vi "sub_pf_localization.vi"(11 "p-val out":T2) -> ()   [LabVIEW 2019]
uses:
  <vilib>/Analysis/Matrix/Datatypes/RealMatrix.ctl
  Ctrl/cmd_common.ctl
  <vilib>/Analysis/baseanly.llb/Real A x B.vi
  <vilib>/ptbypt/NI_PtbyPt.lvlib
  <vilib>/Analysis/NI_AALBase.lvlib
  <vilib>/Analysis/Matrix/NI_Matrix.lvlib
panel:
  out "x":T1 caption="전치 행렬"
  out "px":T1
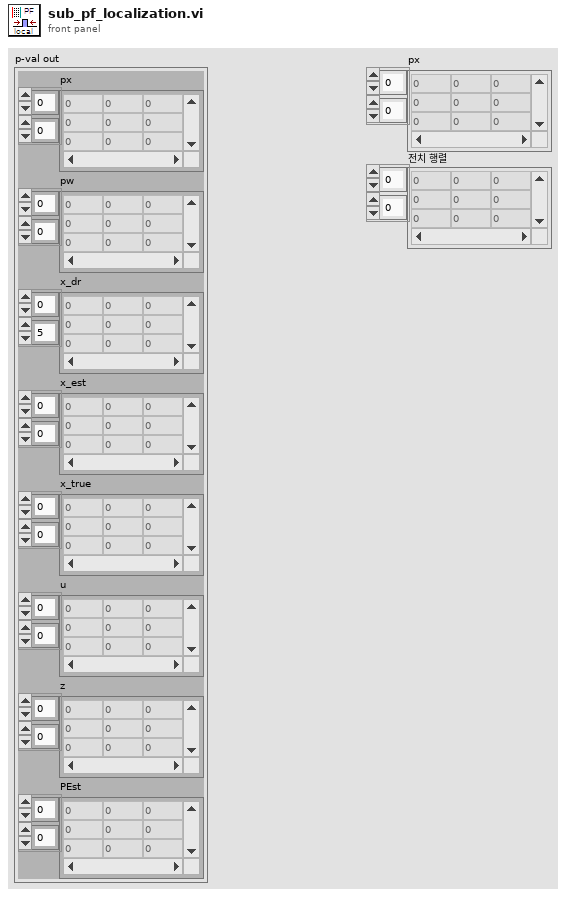
[diagram p1: front panel]
types:
  T1 = typedef "NI_Matrix.lvlib/RealMatrix.ctl" = dbl[][]
  T2 = cluster{"px":T1, "pw":T1, "x_dr":T1, "x_est":T1, "x_true":T1, "u":T1, "z":T1, "PEst":T1}
  T3 = typedef "cmd_common.ctl" = enum16{"read", "write"}
  T4 = cluster{"DT":dbl, "SIM_TIME":dbl, "MAX_RANGE":dbl, "NP":u32, "NTh":u32, "Q":T1, "R":T1, "Q_sim":T1, "R_sim":T1, "rf_id":cluster{"x":dbl, "y":dbl}[]}
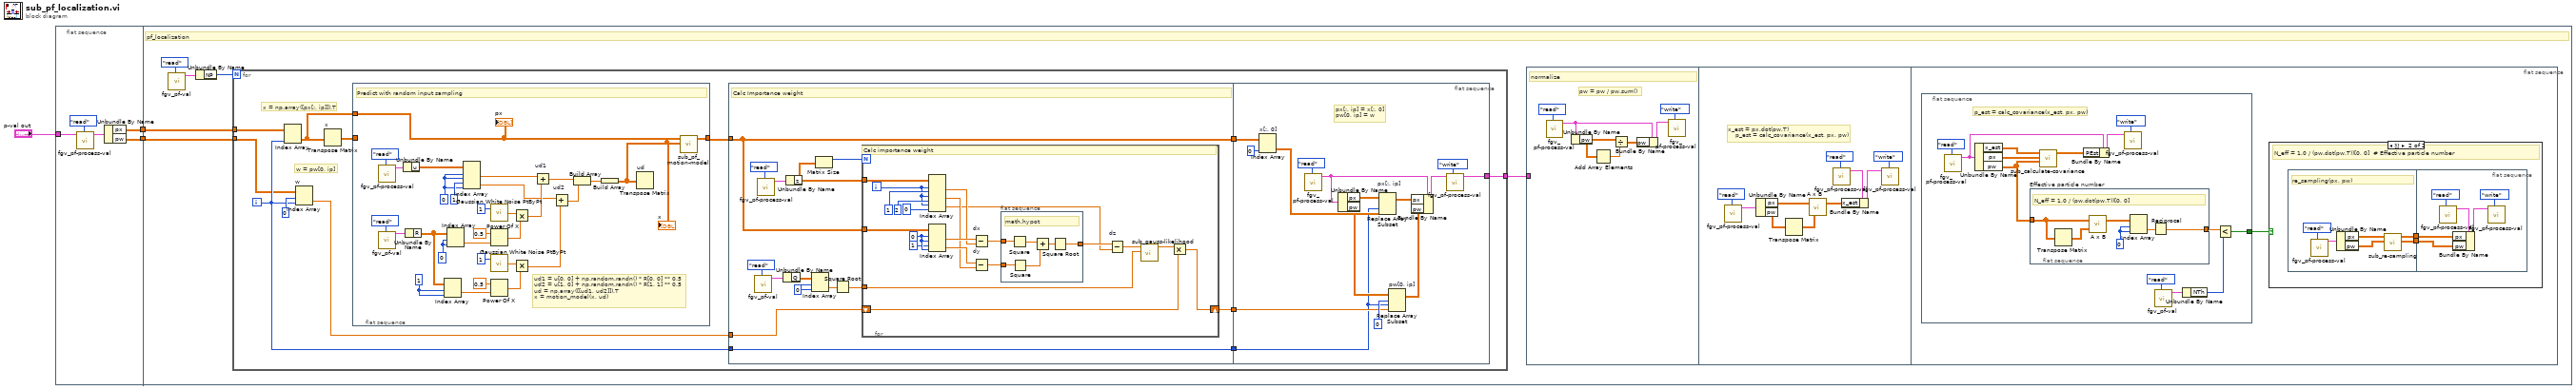
[diagram p0: block diagram]
diagram:
  n1 = flat-sequence {
    tunnel: [w6] -> w3
    tunnel: [w5] -> w2
    tunnel: "p-val out" -> [w4]
    tunnel: w3 -> [w10]
    tunnel: w2 -> [w9]
    frame #0 {
      n2 = call "fgv_pf-process-val.vi"("cmd"=cmd_common."read", "p-val"=w4) -> ("p-val out"=w8:T2)  [unwired: 9 in]
      n3 = Unbundle By Name(w8) -> ("px"=w6:T1, "pw"=w5:T1)
    }
    frame #1 {
      # "pf_localization"
      n4 = call "fgv_pf-val.vi"("cmd"=cmd_common."read") -> ("pf-val out"=w13:T4)  [unwired: 10 in]
      n5 = Unbundle By Name(w13) -> ("NP"=w11:u32)
      n6 = for {
        N: w11 -> [_]
        tunnel: [w71] -> w14
        tunnel: w10 -> [w68]
        tunnel: w9 -> [w67]
        i -> [w70]
        # "x = np.array([px[:, ip]]).T"
        # "w = pw[0, ip]"
        n7 = Index Array(array=w68, index (col)=w70) -> (element=w66:T1)  [unwired: 1 in]
        n8 = Index Array "w"(array=w67, index (row)=0 ("인덱스 (행)"), index (col)=w70) -> (element=w75:dbl)
        n9 = Transpose Matrix "x"(1:w66) -> (0:w69:T1)
        n10 = flat-sequence {
          tunnel: w69 -> [_]
          tunnel: [w80] -> w76
          tunnel: w66 -> [w79]
          frame #0 {
            w88 = 1 ("인덱스 (행)")
            w99 = 0 ("인덱스 (행)")
            w103 = 0 ("인덱스 (행)")
            # "ud1 = u[0, 0] + np.random.randn() * R[0, 0] ** 0.5\nud2 = u[1, 0] + np.random.randn() * R[1, 1] ** 0.5\nud = np.array([[ud1, ud2]]).T\nx = motion_model(x, ud)"
            # "Predict with random input sampling"
            n11 = call "fgv_pf-process-val.vi"("cmd"=cmd_common."read") -> ("p-val out"=w106:T2)  [unwired: 10 in]
            n12 = call "fgv_pf-val.vi"("cmd"=cmd_common."read") -> ("pf-val out"=w100:T4)  [unwired: 10 in]
            n13 = Unbundle By Name(w106) -> ("u"=w105:T1)
            n14 = Unbundle By Name(w100) -> ("R"=w81:T1)
            n15 = Index Array(array=w81, index (row)=w88, index (col)=w88) -> (element=w89:dbl)
            n16 = Index Array(array=w81, index (row)=w99, index (col)=w99) -> (element=w98:dbl)
            n17 = Index Array(array=w105, index (row) #1=w103, index (col) #1=w103, index (row) #2=1 ("인덱스 (행)"), index (col) #2=w103) -> (element #1=w93:dbl, element #2=w86:dbl)
            n18 = call <vilib>:"Gaussian White Noise PtByPt.vi"("standard deviation"=1 ("samples")) -> ("Gaussian white noise"=w95:dbl)  [unwired: 2 in]
            n19 = Power Of X(1:w98, 2:0.5 ("y")) -> (0:w96:dbl)
            n20 = call <vilib>:"Gaussian White Noise PtByPt.vi"("standard deviation"=1 ("samples")) -> ("Gaussian white noise"=w92:dbl)  [unwired: 2 in]
            n21 = Power Of X(1:w89, 2:0.5 ("y")) -> (0:w91:dbl)
            n22 = Multiply(x=w95, y=w96) -> (x*y=w94:dbl)
            n23 = Multiply(x=w92, y=w91) -> (x*y=w85:dbl)
            n24 = Add "ud1"(x=w93, y=w94) -> (x+y=w82:dbl)
            n25 = Add "ud2"(x=w86, y=w85) -> (x+y=w83:dbl)
            n26 = Build Array(w82, w83) -> (w84:dbl[])
            n27 = Build Array(w84) -> (w78:T1)
            "x" <- w78
            n28 = Transpose Matrix "ud"(1:w78) -> ()  [unwired: 1 out]
            n29 = call "sub_pf_motion-model.vi"("u"=w78, "x_true"=w79) -> ("x_true out"=w80:T1)  [unwired: 9 in]
            "px" <- w79
          }
        }
        n30 = flat-sequence {
          tunnel: w76 -> [w109]
          tunnel: w75 -> [w111]
          tunnel: w70 -> [w110]
          tunnel: [w110] -> w74
          tunnel: [w109] -> w73
          tunnel: [w108] -> w72
          tunnel: w72 -> [w153]
          tunnel: w73 -> [w159]
          tunnel: w74 -> [w152]
          tunnel: [w151] -> w71
          frame #0 {
            w114 = 0 ("인덱스 (행)")
            # "Calc Importance weight"
            n31 = call "fgv_pf-val.vi"("cmd"=cmd_common."read") -> ("pf-val out"=w116:T4)  [unwired: 10 in]
            n32 = call "fgv_pf-process-val.vi"("cmd"=cmd_common."read") -> ("p-val out"=w120:T2)  [unwired: 10 in]
            n33 = Unbundle By Name(w116) -> ("Q"=w115:T1)
            n34 = Unbundle By Name(w120) -> ("z"=w118:T1)
            n35 = Index Array(array=w115, index (row)=w114, index (col)=w114) -> (element=w113:dbl)
            n36 = Matrix Size(0:w118) -> (1:w119:i32)  [unwired: 1 out]
            n37 = Square Root(x=w113) -> (sqrt(x)=w112:dbl)
            n38 = for {
              N: w119 -> [_]
              tunnel: w109 -> [w142]
              tunnel: w118 -> [w139]
              tunnel: w112 -> [w126]
              shift-right: [w122] -> w108
              shift-left: w111 -> [w123]
              i -> [w125]
              w141 = 0 ("인덱스 (행)")
              # "Calc importance weight"
              n39 = Index Array(array=w139, index (row) #1=w125, index (col) #1=1 ("인덱스 (열)"), index (row) #2=w125, index (col) #2=2 ("인덱스 (열)"), index (row) #3=w125, index (col) #3=0 ("인덱스 (열)")) -> (element #1=w135:dbl, element #2=w133:dbl, element #3=w128:dbl)
              n40 = Index Array(array=w142, index (row) #1=w141, index (col) #1=w141, index (row) #2=1 ("인덱스 (행)"), index (col) #2=w141) -> (element #1=w136:dbl, element #2=w134:dbl)
              n41 = Subtract "dx"(x=w136, y=w135) -> (x-y=w131:dbl)
              n42 = Subtract "dy"(x=w134, y=w133) -> (x-y=w132:dbl)
              n43 = flat-sequence {
                tunnel: w132 -> [w148]
                tunnel: w131 -> [w147]
                tunnel: [w143] -> w129
                frame #0 {
                  # "math.hypot"
                  n44 = Square(x=w147) -> (x^2=w145:dbl)
                  n45 = Square(x=w148) -> (x^2=w144:dbl)
                  n46 = Add(x=w145, y=w144) -> (x+y=w146:dbl)
                  n47 = Square Root(x=w146) -> (sqrt(x)=w143:dbl)
                }
              }
              n48 = Subtract "dz"(x=w129, y=w128) -> (x-y=w127:dbl)
              n49 = call "sub_gauss-likelihood.vi"("sigma"=w126, "x"=w127) -> ("p"=w124:dbl)  [unwired: 9 in]
              n50 = Multiply ("Multiply.vi")(x=w124, y=w123) -> (x*y=w122:dbl)
            }
          }
          frame #1 {
            # "px[:, ip] = x[:, 0]\npw[0, ip] = w"
            n51 = Index Array "x[:, 0]"(array=w159, index (col)=0) -> (element=w156:T1)  [unwired: 1 in]
            n52 = call "fgv_pf-process-val.vi"("cmd"=cmd_common."read") -> ("p-val out"=w160:T2)  [unwired: 10 in]
            n53 = Unbundle By Name(w160) -> ("px"=w157:T1, "pw"=w155:T1)
            n54 = Replace Array Subset "px[:, ip]"(array=w157, new element=w156, index (col)=w152) -> (w149:T1)  [unwired: 1 in]
            n55 = Replace Array Subset "pw[0, ip]"(array=w155, new element=w153, index (row)=0 ("index (col)"), index (col)=w152) -> (w150:T1)
            n56 = Bundle By Name(cluster=w160, "px"=w149, "pw"=w150) -> (w163:T2)
            n57 = call "fgv_pf-process-val.vi"("cmd"=cmd_common."write", "p-val"=w163) -> ("p-val out"=w151:T2)  [unwired: 9 in]
          }
        }
      }
      n58 = flat-sequence {
        tunnel: w14 -> [_]
        frame #0 {
          # "pw = pw / pw.sum()"
          # "normalize"
          n59 = call "fgv_pf-process-val.vi"("cmd"=cmd_common."read") -> ("p-val out"=w20:T2)  [unwired: 10 in]
          n60 = Unbundle By Name(w20) -> ("pw"=w18:T1)
          n61 = Add Array Elements(numeric array=w18) -> (sum=w17:dbl)
          n62 = Divide(x=w18, y=w17) -> (x/y=w19:T1)
          n63 = Bundle By Name(cluster=w20, "pw"=w19) -> (w21:T2)
          n64 = call "fgv_pf-process-val.vi"("cmd"=cmd_common."write", "p-val"=w21) -> ()  [unwired: 9 in, 1 out]
        }
        frame #1 {
          # "x_est = px.dot(pw.T)\n    p_est = calc_covariance(x_est, px, pw)"
          n65 = call "fgv_pf-process-val.vi"("cmd"=cmd_common."read") -> ("p-val out"=w31:T2)  [unwired: 10 in]
          n66 = Unbundle By Name(w31) -> ("px"=w30:T1, "pw"=w29:T1)
          n67 = Transpose Matrix(1:w29) -> (0:w28:T1)
          n68 = call-poly <vilib>:"A x B.vi"("B"=w28, "A"=w30) -> ("A x B"=w25:T1)  [unwired: 1 out]
          n69 = call "fgv_pf-process-val.vi"("cmd"=cmd_common."read") -> ("p-val out"=w26:T2)  [unwired: 10 in]
          n70 = Bundle By Name(cluster=w26, "x_est"=w25) -> (w27:T2)
          n71 = call "fgv_pf-process-val.vi"("cmd"=cmd_common."write", "p-val"=w27) -> ()  [unwired: 9 in, 1 out]
        }
        frame #2 {
          n72 = flat-sequence {
            tunnel: [w37] -> w32
            frame #0 {
              # "p_est = calc_covariance(x_est, px, pw)"
              n73 = call "fgv_pf-process-val.vi"("cmd"=cmd_common."read") -> ("p-val out"=w35:T2)  [unwired: 10 in]
              n74 = Unbundle By Name(w35) -> ("x_est"=w43:T1, "px"=w44:T1, "pw"=w42:T1)
              n75 = flat-sequence "Effective particle number" {
                tunnel: w42 -> [w51]
                tunnel: [w46] -> w40
                frame #0 {
                  w48 = 0 ("index (row)")
                  # "N_eff = 1.0 / (pw.dot(pw.T))[0, 0]"
                  n76 = Transpose Matrix(1:w51) -> (0:w50:T1)
                  n77 = call-poly <vilib>:"A x B.vi"("B"=w50, "A"=w51) -> ("A x B"=w49:T1)  [unwired: 1 out]
                  n78 = Index Array(array=w49, index (row)=w48, index (col)=w48) -> (element=w47:dbl)
                  n79 = Reciprocal(x=w47) -> (1/x=w46:dbl)
                }
              }
              n80 = call "sub_calculate-covariance.vi"("pw"=w42, "px"=w44, "x_est"=w43) -> ("cov out"=w34:T1)  [unwired: 8 in]
              n81 = Bundle By Name(cluster=w35, "PEst"=w34) -> (w33:T2)
              n82 = call "fgv_pf-process-val.vi"("cmd"=cmd_common."write", "p-val"=w33) -> ()  [unwired: 9 in, 1 out]
              n83 = call "fgv_pf-val.vi"("cmd"=cmd_common."read") -> ("pf-val out"=w39:T4)  [unwired: 10 in]
              n84 = Unbundle By Name(w39) -> ("NTh"=w38:u32)
              n85 = Less?(x=w40, y=w38) -> (x < y?=w37:bool)
            }
          }
          n86 = case shown="참" w32 {
            frame False {
            }
            frame True {
              # "N_eff = 1.0 / (pw.dot(pw.T))[0, 0]  # Effective particle number"
              n87 = flat-sequence {
                tunnel: [w55] -> w53
                tunnel: [w54] -> w52
                tunnel: w53 -> [w63]
                tunnel: w52 -> [w62]
                frame #0 {
                  # "re_sampling(px, pw)"
                  n88 = call "fgv_pf-process-val.vi"("cmd"=cmd_common."read") -> ("p-val out"=w59:T2)  [unwired: 10 in]
                  n89 = Unbundle By Name(w59) -> ("px"=w56:T1, "pw"=w57:T1)
                  n90 = call "sub_re-sampling.vi"("pw"=w57, "px"=w56) -> ("A + c"=w54:T1, "Real Matrix"=w55:T1)  [unwired: 8 in]
                }
                frame #1 {
                  n91 = call "fgv_pf-process-val.vi"("cmd"=cmd_common."read") -> ("p-val out"=w65:T2)  [unwired: 10 in]
                  n92 = Bundle By Name(cluster=w65, "px"=w63, "pw"=w62) -> (w64:T2)
                  n93 = call "fgv_pf-process-val.vi"("cmd"=cmd_common."write", "p-val"=w64) -> ()  [unwired: 9 in, 1 out]
                }
              }
            }
          }
        }
      }
    }
  }
